vi "getLedRefnum.vi"(8 "error in (no error)":errorcluster, 11 "LED in":refnum<class "LED.lvclass">) -> (0 "error out":errorcluster, 2 "LED Refnum":refnum<vi>, 3 "LED out":refnum<class "LED.lvclass">)   [LabVIEW 2020, in "LED.lvclass"]
uses:
  LED.lvclass
  LED.lvclass/LED.ctl
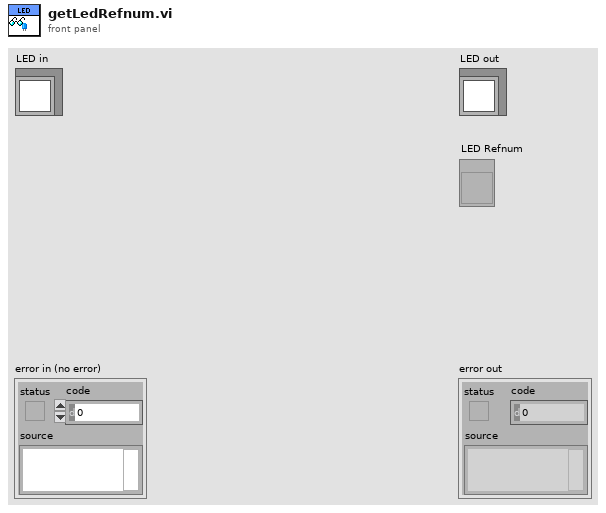
[diagram p1: front panel]
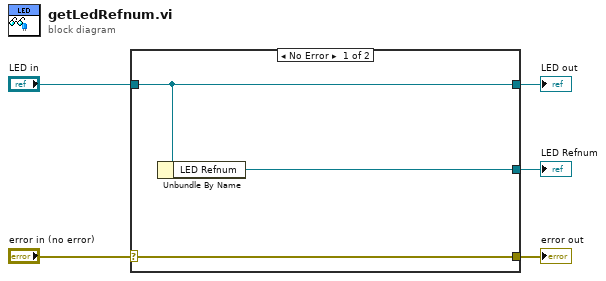
[diagram p0: block diagram]
diagram:
  n1 = case shown="No Error" "error in (no error)" {
    selector: "error in (no error)" -> [w8 w9]
    tunnel: [w8 w9] -> w4
    tunnel: [w7 w10] -> w2
    tunnel: "LED in" -> [w7 w10]
    tunnel: [w6 _] -> w1
    frame No Error {
      n2 = Unbundle By Name(w7) -> ("LED Refnum"=w6:refnum<vi>)
    }
    frame Error {
    }
  }
  "error out" <- w4
  "LED out" <- w2
  "LED Refnum" <- w1
